vi "Ohrev.vi"() -> ()   [LabVIEW 2016]
panel:
  in  "Boolean":bool
  out "Výøivka 2":bool
  out "Výøivka 1":bool
  in  "Ohøev zapnout":bool
  out "Teplota výøivky 1":dbl(slide) scale=0.0..100.0
  # "Teplota výøivek"
  # "Signalizace výøivek"
  # "Signalizace ohøevu"
  # "Aktuální teplota-Když je vyšší než 32, vypnout ohøev\n                              Když je nižší, než 28, zapnout ohøev"
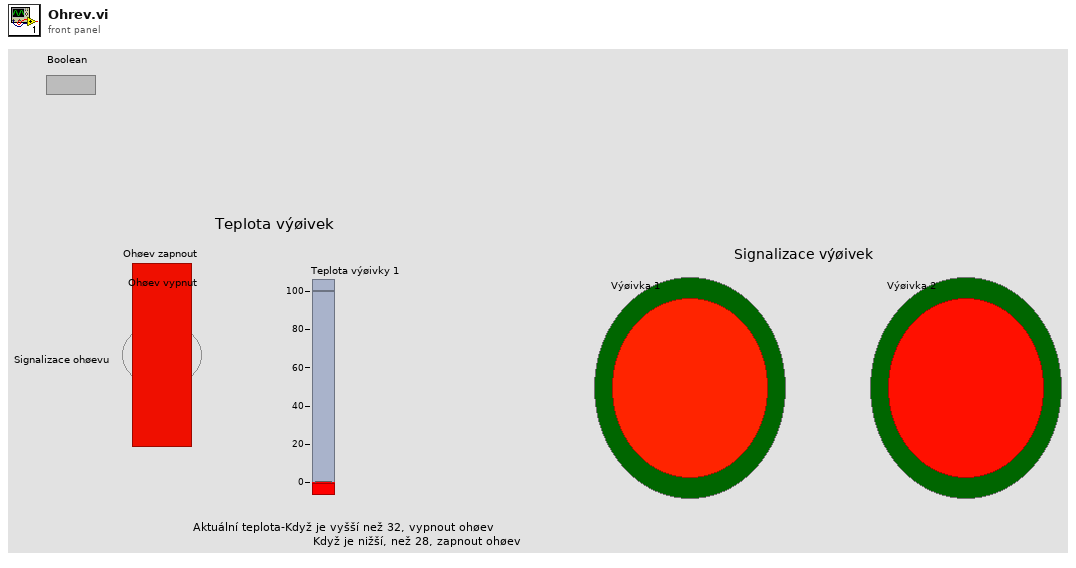
[diagram p1: front panel]
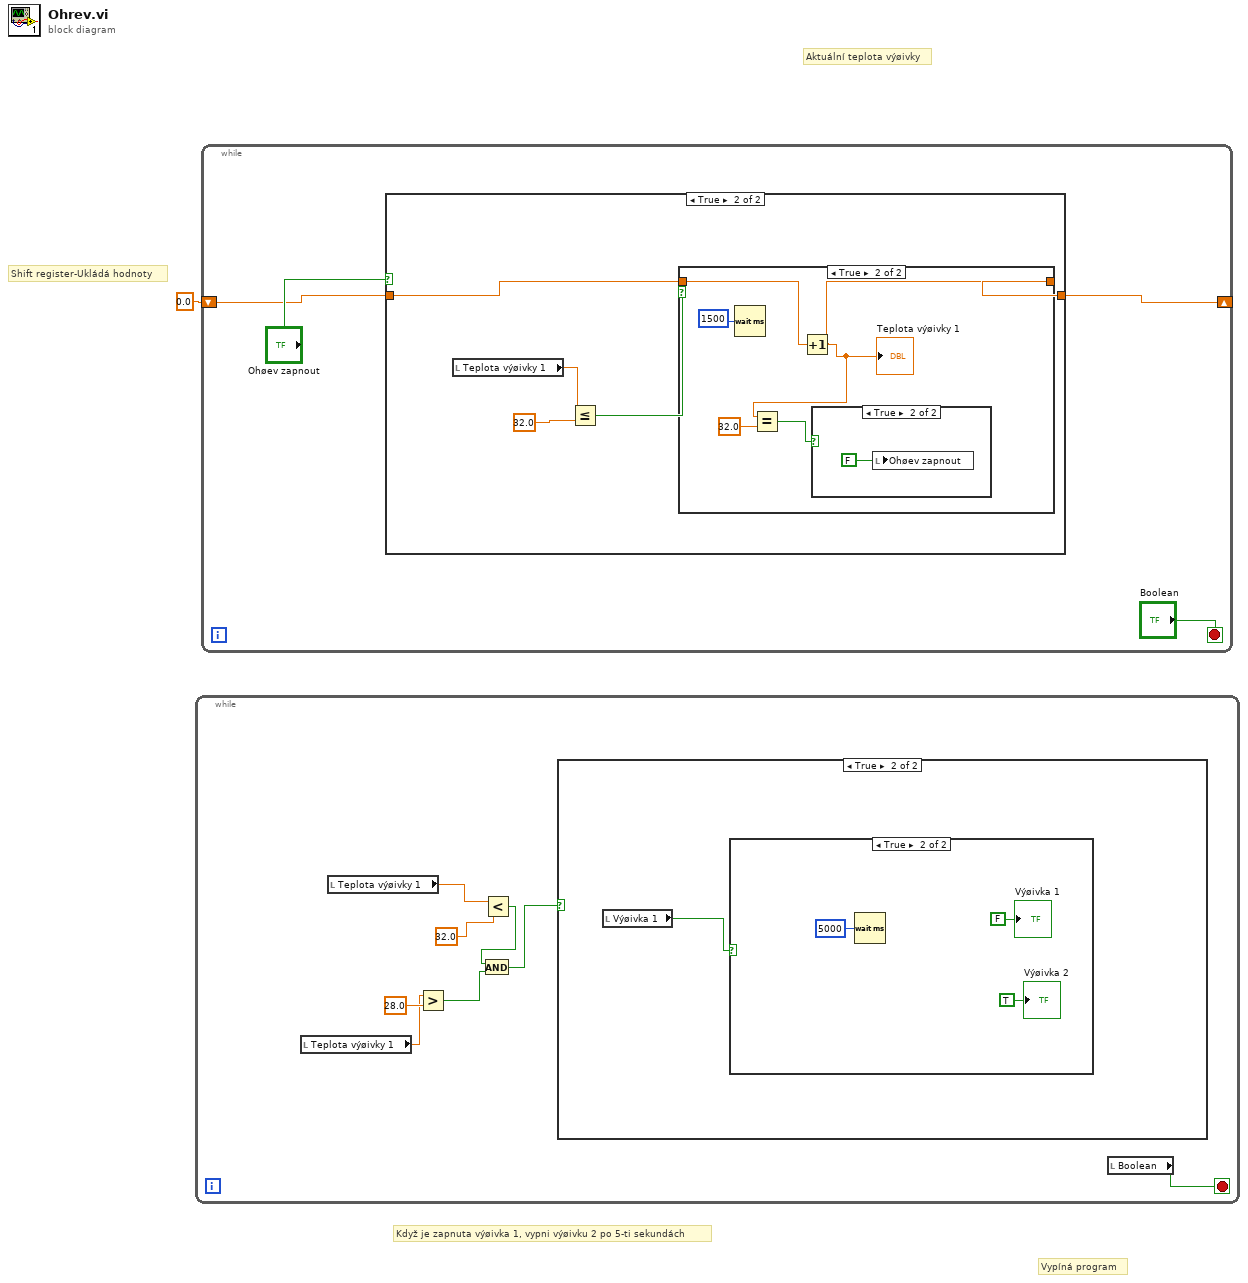
[diagram p0: block diagram]
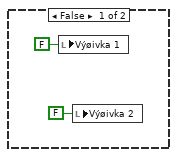
[diagram p2: hidden frame]
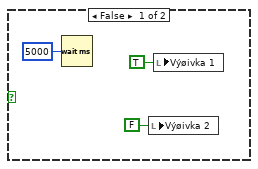
[diagram p3: hidden frame]
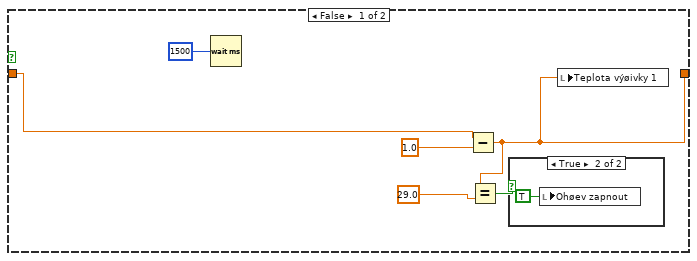
[diagram p4: hidden frame]
diagram:
  # "Vypíná program"
  # "Když je zapnuta výøivka 1, vypni výøivku 2 po 5-ti sekundách"
  # "Aktuální teplota výøivky"
  # "Shift register-Ukládá hodnoty"
  n1 = while {
    stop <- w2 stop-if-true
    n2 = local read "Teplota výøivky 1"() -> (w6:dbl)
    n3 = local read "Teplota výøivky 1"() -> (w9:dbl)
    n4 = Greater?(x=w6, y=28.0) -> (0:w4:bool)
    n5 = Less?(x=w9, y=32.0) -> (x < y?=w5:bool)
    n6 = And(x=w5, y=w4) -> (x .and. y?=w3:bool)
    n7 = case shown="True" w3 {
      frame False {
        n8 = local write "Výøivka 1"(FALSE ("Výøivka 1")) -> ()
        n9 = local write "Výøivka 2"(FALSE ("Výøivka 2")) -> ()
      }
      frame True {
        n10 = local read "Výøivka 1"() -> (w12:bool)
        n11 = case shown="True" w12 {
          frame False {
            n12 = Wait (ms)(milliseconds to wait=u32 5000) -> ()  [unwired: 1 out]
            n13 = local write "Výøivka 2"(FALSE ("Výøivka 2")) -> ()
            n14 = local write "Výøivka 1"(TRUE ("Výøivka 1")) -> ()
          }
          frame True {
            n15 = Wait (ms)(milliseconds to wait=u32 5000) -> ()  [unwired: 1 out]
            "Výøivka 1" <- FALSE ("Výøivka 1")
            "Výøivka 2" <- TRUE ("Výøivka 2")
          }
        }
      }
    }
    n16 = local read "Boolean"() -> (w2:bool)
  }
  n17 = while {
    shift-right: [w21] -> _
    shift-left: 0.0 -> [w20]
    stop <- "Boolean" stop-if-true
    n18 = case shown="True" "Ohøev zapnout" {
      tunnel: [w25 w31] -> w21
      tunnel: w20 -> [w24 w30]
      frame False {
        n19 = Wait (ms)(milliseconds to wait=u32 1500) -> ()  [unwired: 1 out]
        n20 = Subtract(x=w24, y=1.0) -> (x-y=w25:dbl)
        n21 = Equal?(x=w25, y=29.0) -> (x = y?=w26:bool)
        n22 = case shown="True" w26 {
          frame False {
          }
          frame True {
            n23 = local write "Ohøev zapnout"(TRUE ("Ohøev zapnout")) -> ()
          }
        }
        n24 = local write "Teplota výøivky 1"(w25) -> ()
      }
      frame True {
        n25 = local read "Teplota výøivky 1"() -> (w34:dbl)
        n26 = Less Or Equal?(x=w34, y=32.0) -> (x <= y?=w32:bool)
        n27 = case shown="True" w32 {
          tunnel: [w35 w38] -> w31
          tunnel: w30 -> [w35 w39]
          frame False {
          }
          frame True {
            n28 = Wait (ms)(milliseconds to wait=u32 1500) -> ()  [unwired: 1 out]
            n29 = Increment(x=w39) -> (x+1=w38:dbl)
            "Teplota výøivky 1" <- w38
            n30 = Equal?(x=w38, y=32.0) -> (x = y?=w36:bool)
            n31 = case shown="True" w36 {
              frame False {
              }
              frame True {
                n32 = local write "Ohøev zapnout"(FALSE ("Ohøev zapnout")) -> ()
              }
            }
          }
        }
      }
    }
  }
